vi "I2C Read.vi"(5 "EOF":T1, 6 "Timeout (1000 ms)":u16=1000, 7 "I2C Channel (0)":u8, 8 "Error In":errorcluster, 9 "Bytes To Read":u8, 10 "I2C Slave Address":u8, 11 "LINX Device Config":T2) -> (0 "Error Out":errorcluster, 2 "Data":u8[](array[numeric]), 3 "LINX Device Config":T2)   [LabVIEW 2014, in "LMH-LINX.lvlib" / "Device.lvlib"]
uses:
  <vilib>/MakerHub/LINX/Private/Device/Device.lvlib
  <vilib>/MakerHub/LINX/Private/Device/Type Defs/LINX Device Config.ctl
  <vilib>/MakerHub/LINX/Private/Type Defs/Interface.ctl
  <vilib>/MakerHub/LINX/Private/Device/Type Defs/TCP Config.ctl
  <vilib>/MakerHub/LINX/Private/Device/Type Defs/Channels.ctl
  <vilib>/MakerHub/LINX/Private/Type Defs/Peripherals/I2C/EOF.ctl
  <vilib>/MakerHub/LINX/Private/Type Defs/Error Type.ctl
  <vilib>/MakerHub/LINX/LMH-LINX.lvlib
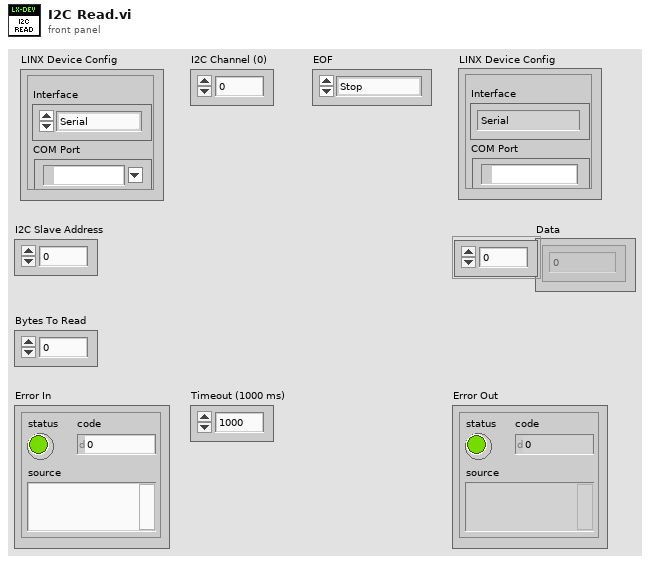
[diagram p1: front panel]
types:
  T1 = typedef "LMH-LINX.lvlib/EOF.ctl" = enum8{"Stop", "Restart", "Restart No Stop", "No Stop"}
  T2 = typedef "LMH-LINX.lvlib/Device.lvlib/LINX Device Config.ctl" = cluster{"Interface":T3, "COM Port":refnum<visa-resource-name>, "TCP Configuration":T4, "Device Family":u8, "Device ID":u8, "Device Name":string, "TCP Ref":refnum<k5>, "Channels":T5}
  T3 = typedef "LMH-LINX.lvlib/Interface.ctl" = enum16{"Serial", "TCP"}
  T4 = typedef "LMH-LINX.lvlib/Device.lvlib/TCP Config.ctl" = cluster{"IP Address":string, "Port":u16}
  T5 = typedef "LMH-LINX.lvlib/Channels.ctl" = cluster{"DI":u8[], "DO":u8[], "AI":u8[], "AO":u8[], "PWM":u8[], "QE":u8[], "UART":u8[], "I2C 2":u8[], "SPI":u8[], "CAN":u8[], "Servo":u8[], "AI Ref (V)":dbl, "AI Resolution (Bits)":u8, "AO Ref (V)":dbl, "AO Resolution (Bits)":u8}
  T6 = typedef "LMH-LINX.lvlib/Error Type.ctl" = enum16{"Unknown", "Timeout", "Corrupt Return Packet", "Unable To Connect", "Command Not Supported", "Channel DNE", "Invalid COM Config", "Firmware Version Mismatch", "myRIO Support", "CMD Specific Error", "Local IO Not Supported"}
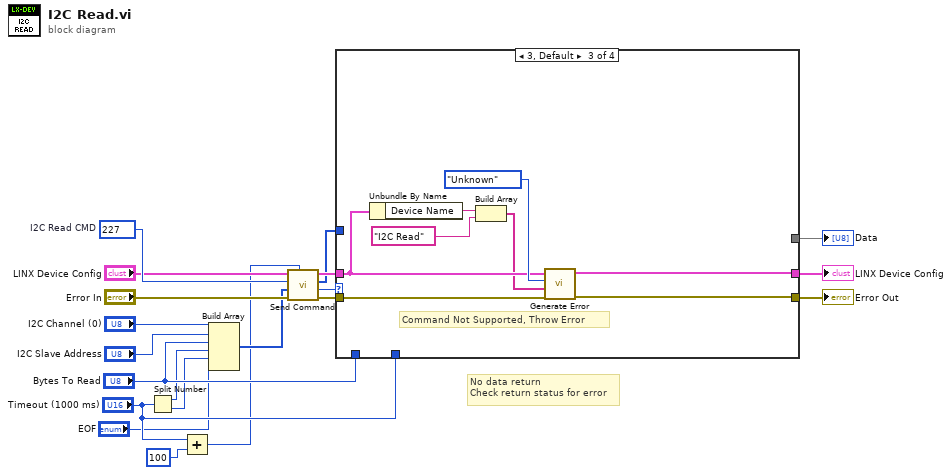
[diagram p0: block diagram]
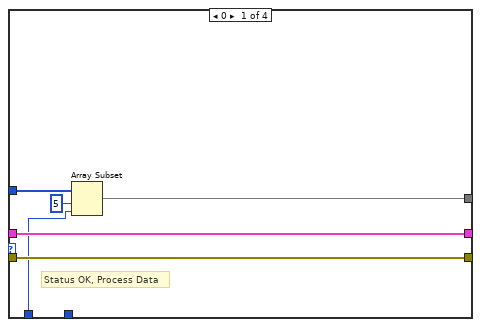
[diagram p2: hidden frame]
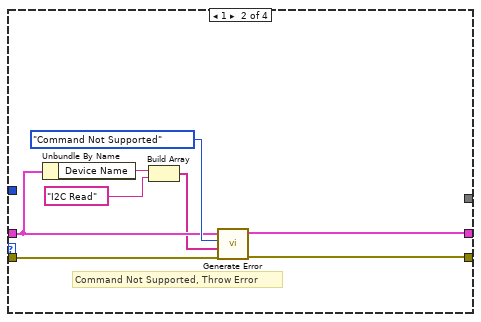
[diagram p3: hidden frame]
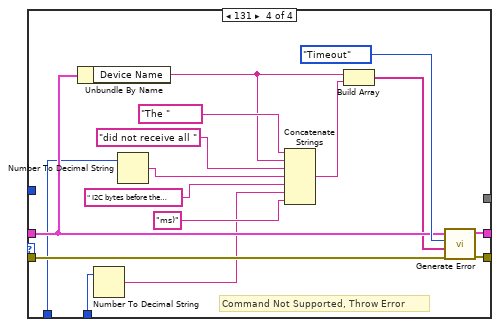
[diagram p4: hidden frame]
diagram:
  w19 = u16 227  # I2C Read CMD
  # "No data return\nCheck return status for error"
  n1 = Split Number(x="Timeout (1000 ms)") -> (hi(x)=w7:u8, lo(x)=w6:u8)
  n2 = Add(x="Timeout (1000 ms)", y=u16 100) -> (x+y=w2:u16)
  n3 = Build Array("I2C Channel (0)", "I2C Slave Address", "Bytes To Read", w7, w6, "EOF") -> (w12:u8[])
  n4 = call <vilib>:"Send Command.vi"("Timeout (100 ms)"=w2, "Error In"="Error In", "ARGS"=w12, "CMD"=w19, "LINX Device Config"="LINX Device Config") -> ("Error Out"=w14:errorcluster, "Status"=w9:u8, "Response"=w13:u8[], "LINX Device Config"=w16:T2)  [unwired: 3 in]
  n5 = case shown="3, Default" w9 {
    tunnel: [w26 w32 w40 w56] -> w17
    tunnel: w16 -> [w26 w30 w38 w54]
    tunnel: [w25 w33 w41 w57] -> w15
    tunnel: w14 -> [w25 w34 w42 w58]
    tunnel: w13 -> [w24 _ _ _]
    tunnel: "Bytes To Read" -> [w22 _ _ w47]
    tunnel: "Timeout (1000 ms)" -> [_ _ _ w44]
    tunnel: [w21 _ _ _] -> w5
    frame 0 {
      # "Status OK, Process Data"
      n6 = Array Subset(array=w24, index=5, length=w22) -> (w21:u8[])
    }
    frame 1 {
      # "Command Not Supported, Throw Error"
      n7 = Unbundle By Name(w30) -> ("Device Name"=w29:string)
      n8 = Build Array(w29, "I2C Read") -> (w27:string[])
      n9 = call <vilib>:"Generate Error.vi"("Error In"=w34, "Arguments"=w27, "Error Type"=Error_Type."Command Not Supported", "LINX Device Config"=w30) -> ("Error Out"=w33:errorcluster, "Dup LINX Device Config"=w32:T2)  [unwired: 6 in]
    }
    frame 3, Default {
      # "Command Not Supported, Throw Error"
      n10 = Unbundle By Name(w38) -> ("Device Name"=w37:string)
      n11 = Build Array(w37, "I2C Read") -> (w35:string[])
      n12 = call <vilib>:"Generate Error.vi"("Error In"=w42, "Arguments"=w35, "Error Type"=Error_Type."Unknown", "LINX Device Config"=w38) -> ("Error Out"=w41:errorcluster, "Dup LINX Device Config"=w40:T2)  [unwired: 6 in]
    }
    frame 131 {
      # "Command Not Supported, Throw Error"
      n13 = Unbundle By Name(w54) -> ("Device Name"=w48:string)
      n14 = Number To Decimal String(number=w44) -> (decimal integer string=w43:string)  [unwired: 1 in]
      n15 = Number To Decimal String(number=w47) -> (decimal integer string=w45:string)  [unwired: 1 in]
      n16 = Concatenate Strings("The ", w48, "did not receive all " ("string"), w45, " I2C bytes before the specified tiemout (" ("string"), w43, "ms)" ("string")) -> (w49:string)
      n17 = Build Array(w48, w49) -> (w53:string[])
      n18 = call <vilib>:"Generate Error.vi"("Error In"=w58, "Arguments"=w53, "Error Type"=Error_Type."Timeout", "LINX Device Config"=w54) -> ("Error Out"=w57:errorcluster, "Dup LINX Device Config"=w56:T2)  [unwired: 6 in]
    }
  }
  "Error Out" <- w15
  "LINX Device Config" <- w17
  "Data" <- w5
